vi "Not.vi"(11 "Node In":refnum<class "bt_Node.lvclass">) -> (3 "Node":refnum<class "bt_Node.lvclass">)   [LabVIEW 2021, in "BT.lvlib"]
uses:
  BT.lvlib
  Support/Nodes/abs_Node/bt_Node.lvclass
  Support/Nodes/Decorators/Not/bt_Not.lvclass
  C:/Users/Tim/Documents/GitHub/LV_Behaviour_Tree/Source/Support/Nodes/Decorators/abs_Decorator/abs_Decorator.lvclass
  C:/Users/Tim/Documents/GitHub/LV_Behaviour_Tree/Source/Support/Nodes/abs_Node/bt_Node.lvclass
  Support/Nodes/Decorators/Support/Decorator/bt_Decorator.lvclass/bt_Decorator.ctl
  Support/Nodes/Decorators/Support/Decorator/Properties/Write Node.vi
  C:/Users/Tim/Documents/GitHub/LV_Behaviour_Tree/Source/Support/Nodes/Decorators/Support/Decorator/bt_Decorator.lvclass
  C:/Users/Tim/Documents/GitHub/LV_Behaviour_Tree/Source/Support/Nodes/Decorators/Not/bt_Not.lvclass
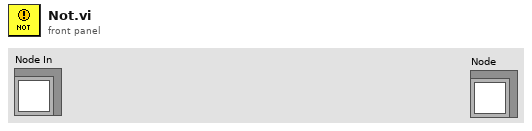
[diagram p1: front panel]
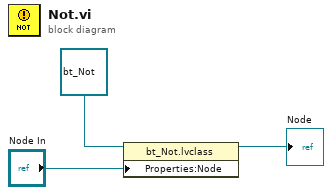
[diagram p0: block diagram]
diagram:
  n1 = property class="bt_Not.lvclass"(reference=refnum<class "bt_Not.lvclass"> refnum ("BT.lvlib:Not.lvclass"), "Properties:Node"="Node In") -> (reference out=→"Node":refnum<class "bt_Not.lvclass">)  [unwired: 1 in, 1 out]
